vi "CSM-FileSync.vi"(5 "Name(FileSync)":string="FileSync", 7 "Protocol.lvclass":refnum<class "Protocol.lvclass">, 11 "FileSync Configuration":T1={"MonitoringFolder"=path "_sync/Monitoring", "BackupFolder"=path "_sync/backup", "autostart"=TRUE, "Backup"=FALSE}) -> (0 "error out":errorcluster)   [LabVIEW 2020, in "CSM-FileSync.lvlib"]
doc: "------------- lvcsm -------------\n[CSMStates]\nItem 0 = \"Idle\"\nItem 1 = \"Timeout\"\nItem 2 = \"Initialize Core Data\"\nItem 3 = \"Error Handler\"\nItem 4 = \"VI Reference\"\nItem 5 = \"Exit\"\nItem 6 = \"Data: Initialize\"\nItem 7 = \"Data: Load Configuration\"\nItem 8 = \"Data: Save Configuration\"\nItem 9 = \"Data: Cleanup\"\nItem 10 = \"UI: Initialize\"\nItem 11 = \"UI: Publish Status\"\nItem 12 = \"Macro: Initialize\"\nItem 13 = \"Macro: FileSync Protocol Connect\"\nItem 14 = \"Macro: Check Is Still Alive\"\nItem 15 = \"Macro: FileSync Routines\"\nItem 16 = \"Macro: FileSync Protocol Disconnect\"\nItem 17 = \"Macro: Exit\"\nItem 18 = \"API: Start\"\nItem 19 = \"API: Stop\"\nItem 20 = \"FileSync: Load Configuration\"\nItem 21 = \"FileSync: Try to Connect\"\nItem 22 = \"FileSync: Status Check\"\nItem 23 = \"FileSync: Close Connection\"\nItem 24 = \"FileSync: Cleanup Protocol\"\nItem 25 = \"FileSyncRoutine: Create Dir if Not Exist\"\nItem 26 = \"FileSyncRoutine: List Files\"\nItem 27 = \"FileSyncRoutine: Pick Uploading File\"\nItem 28 = \"FileSyncRoutine: Upload\"\nItem 29 = \"FileSyncRoutine: Move File to Backup Folder\"\nItem 30 = \"FileSyncRoutine: Remove Empty Container Folder\"\n\n[CSMStatus]\nItem 0 = \"Status Change@UI: Publish Status\"\nItem 1 = \"Uploading List Change@UI: Publish Status\""
uses:
  CSM-FileSync.lvlib
  Protocol/Base/Protocol.lvclass
  Protocol/Base/Def-FileSyncConfig.ctl
  c11ad69d-c218-40bd-9883-d3361c9d07ec.vi
  4f3a877e-8c3a-40cf-89f4-fda6eeae6ffa.vi
  d714c97a-ade9-4c5a-b010-05319b638c8a.vi
  16b40464-5854-4f01-88e3-2a837e9228b3.vi
  16b40464-5854-4f01-88e3-2a837e9228b3.vi/eb2405bd-5b2e-436b-9bb3-692ecf4a9268.vi
  16b40464-5854-4f01-88e3-2a837e9228b3.vi/c8ad12e3-5e6d-40e1-92e0-1426ef45ec41.vi
  16b40464-5854-4f01-88e3-2a837e9228b3.vi/effcbc1a-e97c-42d4-b61f-d821de102707.vi
  <userlib>/_NEVSTOP/Communicable State Machine(CSM)/addons/MassData-Parameter/_support/FGV-MassData(lvlibp).vi
  <userlib>/_NEVSTOP/Communicable State Machine(CSM)/_Polymophic/Add State(s) to Queue By BOOL(Element).vi
  <userlib>/_NEVSTOP/Communicable State Machine(CSM)/_Polymophic/Build Status Broadcast Message.vi
  <userlib>/_NEVSTOP/Communicable State Machine(CSM)/AdvanceAPI/CSM - Set Module Attribute.vi
  <userlib>/_NEVSTOP/Communicable State Machine(CSM)/addons/API-String-Arugments-Support/_Support/Data To API String Arguments.vi
  <userlib>/_NEVSTOP/Communicable State Machine(CSM)/Communicable State Machine.lvlib
  <userlib>/_NEVSTOP/Communicable State Machine(CSM)/addons/Logger/CSM File Logger.lvlib
  <userlib>/_NEVSTOP/Communicable State Machine(CSM)/addons/Loop-Support/CSM Loop Support.lvlib
  <userlib>/_NEVSTOP/Communicable State Machine(CSM)/addons/MassData-Parameter/CSM MassData Parameter Support.lvlib
panel:
  out "State History":string
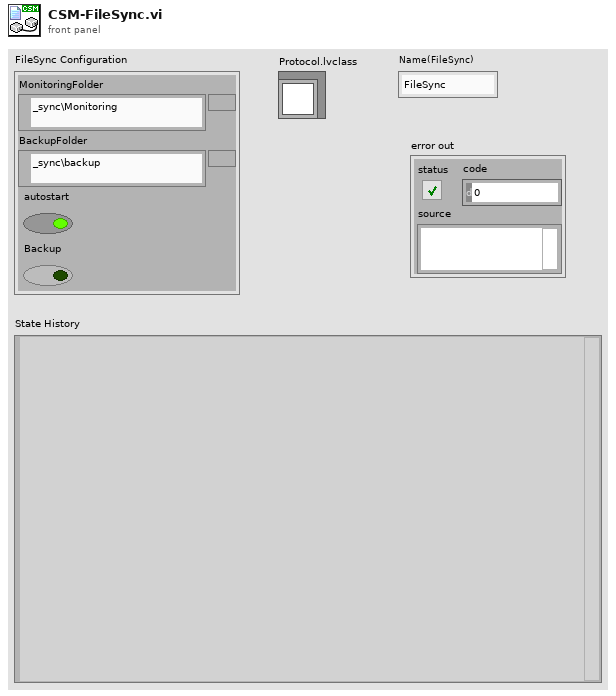
[diagram p1: front panel]
types:
  T1 = typedef "CSM-FileSync.lvlib/Protocol.lvclass/Def-FileSyncConfig.ctl" = cluster{"MonitoringFolder":path, "BackupFolder":path, "autostart":bool, "Backup":bool}
  T2 = enum32{"Invalid", "Standard", "Closed", "Hidden", "Minimized", "Maximized"}
  T3 = enum32{"invalid app kind", "Development System", "Run Time System", "Student Edition", "Embedded LabVIEW", "Evaluation", "Custom"}
  T4 = cluster{"Upload List":path[], "UploadingFile":path}
  T5 = typedef "Communicable State Machine.lvlib/_CSM_Response Source Message.ctl" = cluster{"‘State":string, "’Arguments":string, "’Error":errorcluster}
  T6 = cluster{"Core":cluster{"Current VI Reference":refnum<vi>, "Close Panel on Exit?":bool}, "Configuration":T1, "FileSync Status":cluster{"Connected":bool}, "Upload List":path[], "Temp:UploadingFile":path}
  T7 = cluster{"Current VI Reference":refnum<vi>, "Close Panel on Exit?":bool}
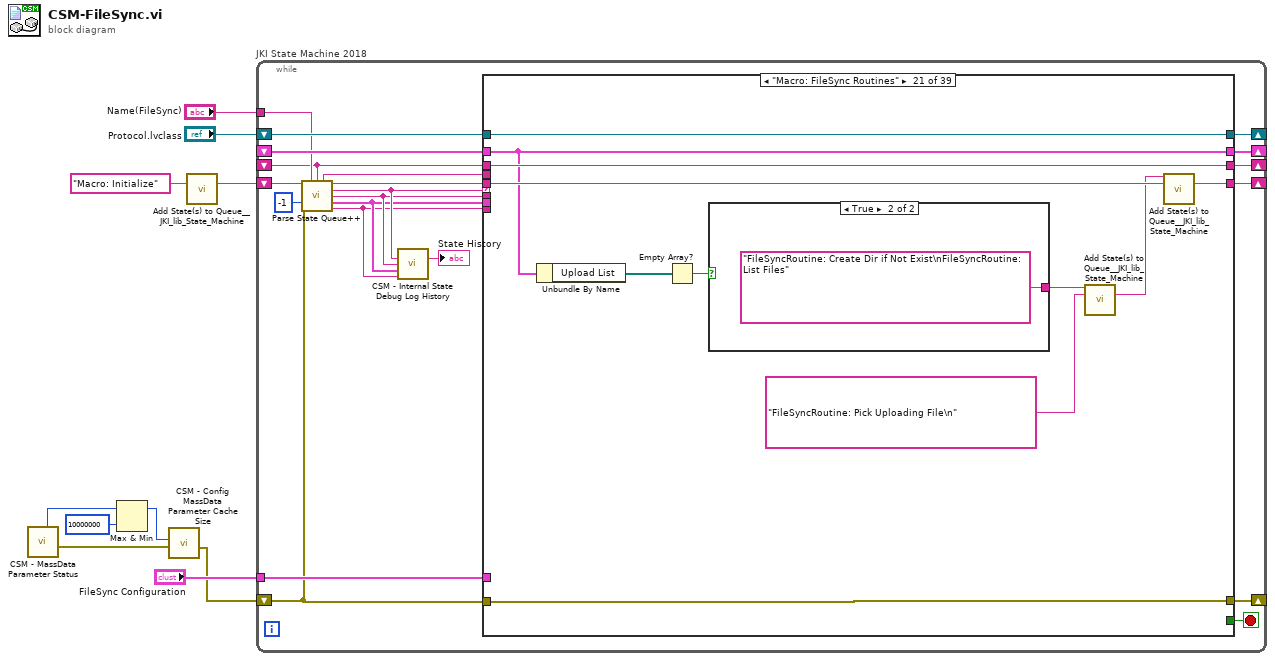
[diagram p0: block diagram]
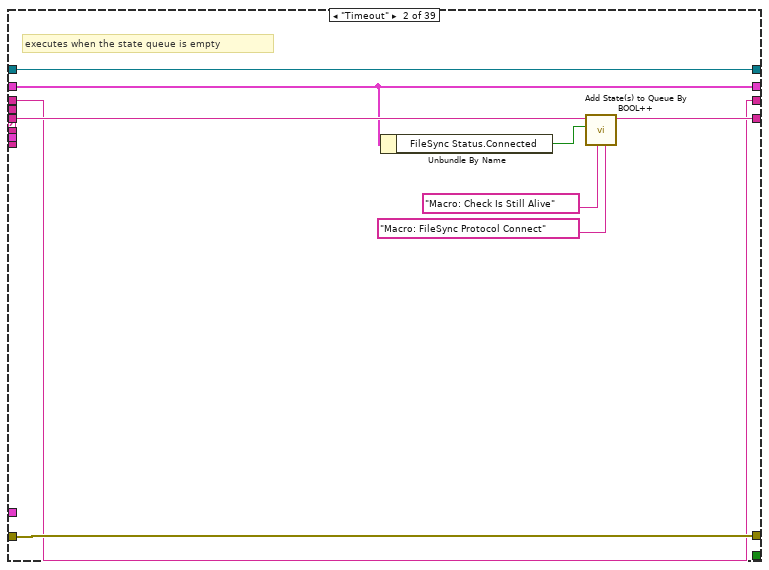
[diagram p3: hidden frame]
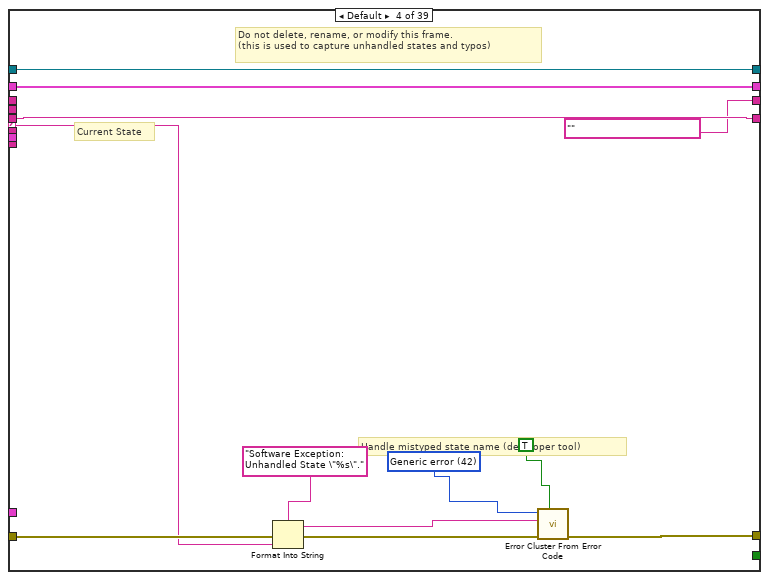
[diagram p5: hidden frame]
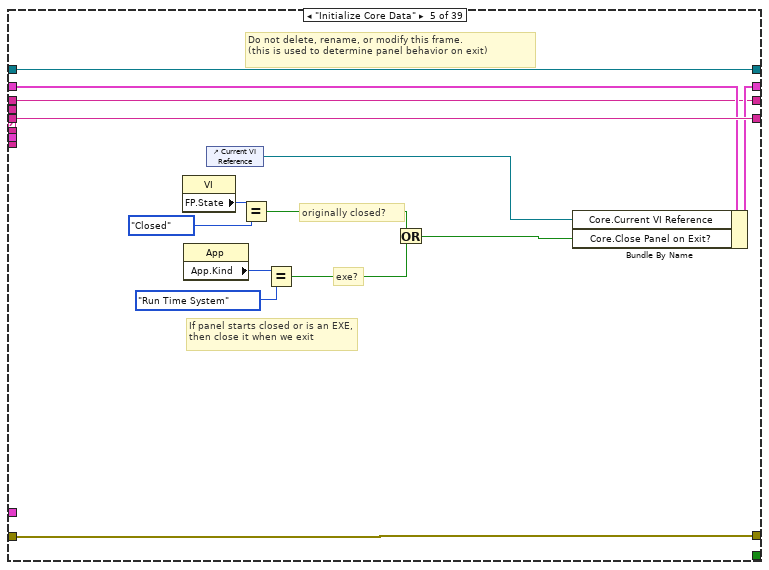
[diagram p6: hidden frame]
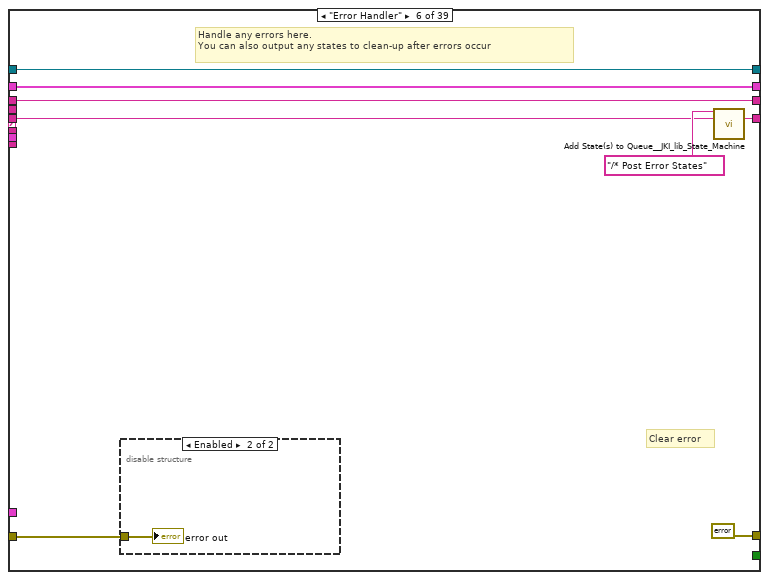
[diagram p7: hidden frame]
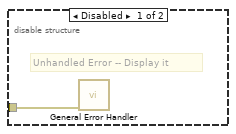
[diagram p8: hidden frame]
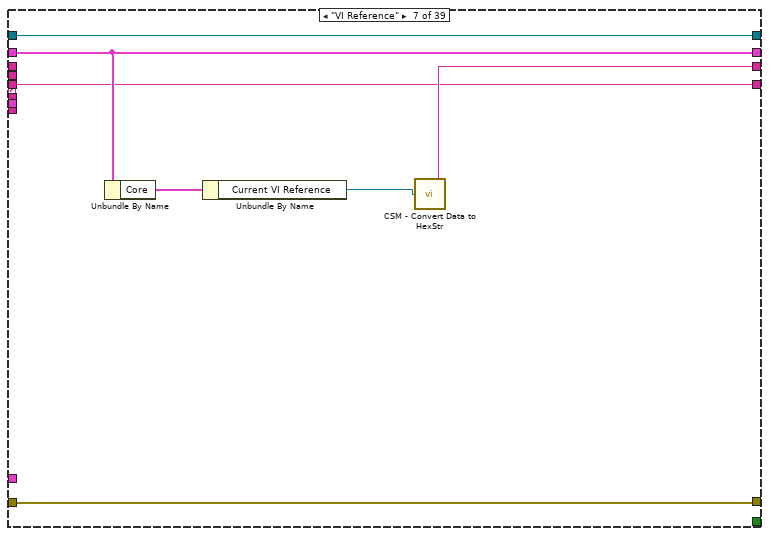
[diagram p9: hidden frame]
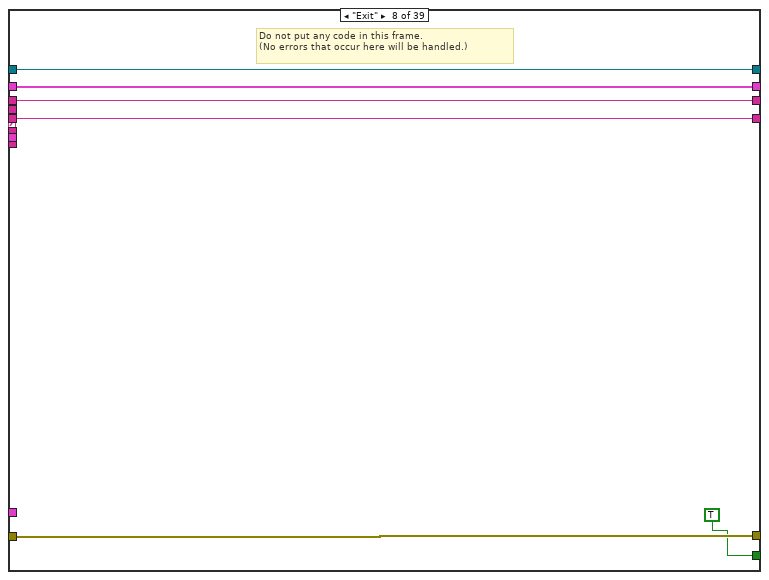
[diagram p10: hidden frame]
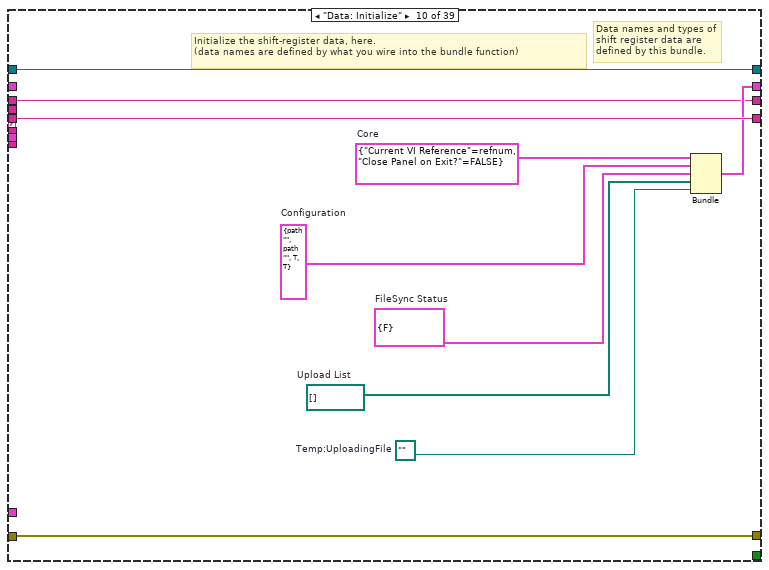
[diagram p12: hidden frame]
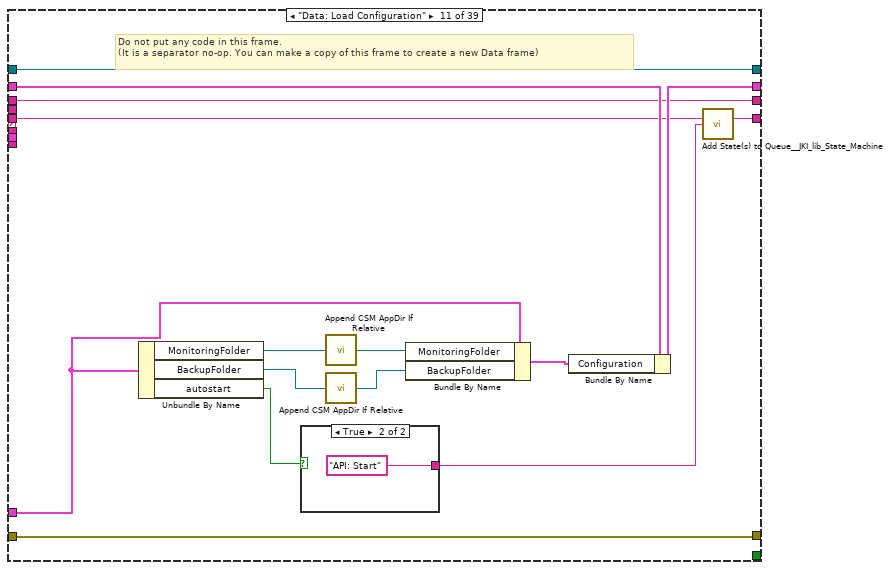
[diagram p13: hidden frame]
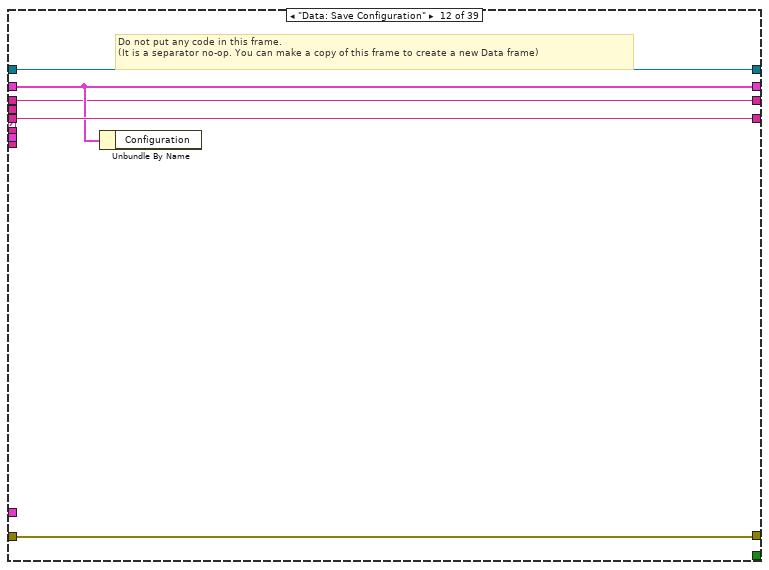
[diagram p15: hidden frame]
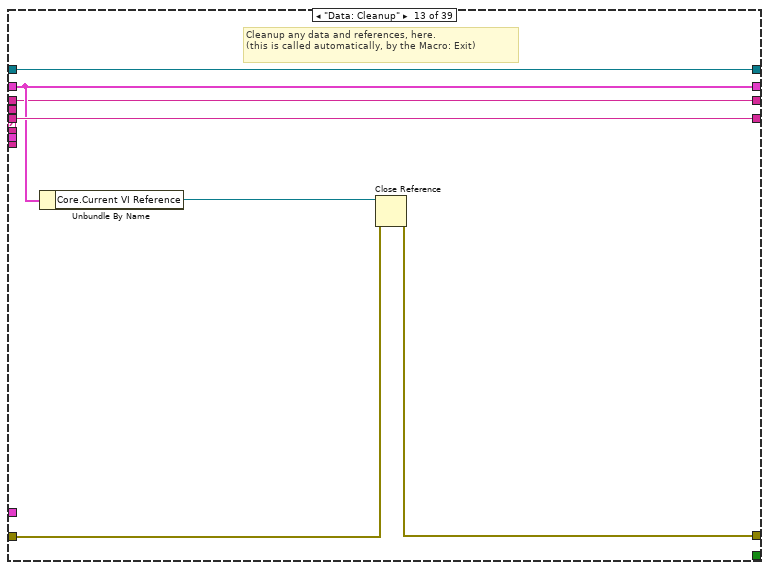
[diagram p16: hidden frame]
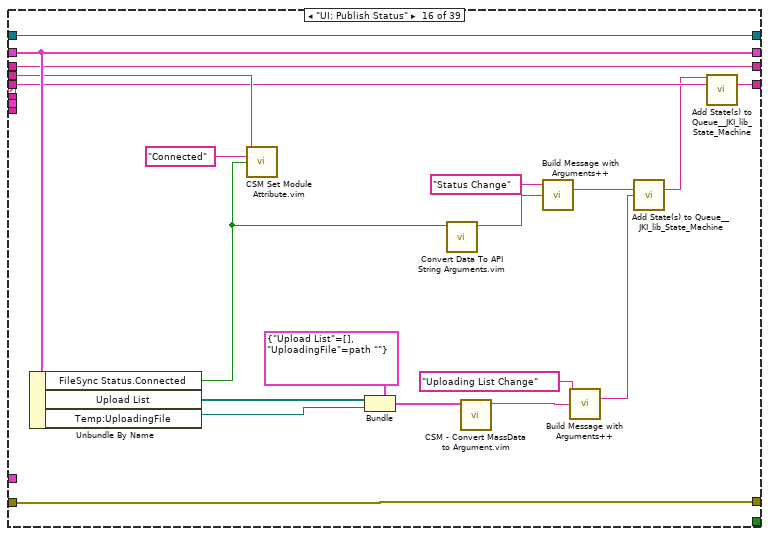
[diagram p19: hidden frame]
diagram:
  n1 = call <userlib>:"CSM - MassData Parameter Status.vi"() -> ("Error out"=w5:errorcluster, "Cache Size"=w2:i32)  [unwired: 7 in, 2 out]
  n2 = Max & Min(x=w2, y=10000000) -> (max(x,y)=w3:i32)  [unwired: 1 out]
  n3 = call <userlib>:"CSM - Config MassData Parameter Cache Size.vi"("Error in"=w5, "Size (50M)"=w3) -> ("Error out"=w4:errorcluster)  [unwired: 9 in]
  n4 = call <vilib>:"Add State(s) to Queue__JKI_lib_State_Machine.vi"("State(s) in (\"\")"="Macro: Initialize") -> ("States Out"=w10:string)  [unwired: 14 in]
  n5 = while "JKI State Machine 2018" {
    shift-right: [w28] -> _
    shift-left: _ -> [w27]
    shift-right: [w31] -> _
    shift-left: w4 -> [w22]
    shift-right: [w30] -> _
    shift-left: w10 -> [w23]
    shift-right: [w25] -> _
    shift-left: "Protocol.lvclass" -> [w26]
    tunnel: "FileSync Configuration" -> [w24]
    shift-right: [w20] -> _
    shift-left: _ -> [w17]
    tunnel: "Name(FileSync)" -> [w19]
    stop <- w29 stop-if-true
    n6 = call <userlib>:"Parse State Queue++.vi"("State Queue"=w23, "Name (\"\" to Use UUID)"=w19, "Response Arguments"=w17, "Previous Error"=w22, "Dequeue (1 ms)"=-1 ("Dequeue Timeout(1ms)")) -> ("Name Used"=w18:string, "Remaining States"=w21:string, "Current State"=w15:string, "Arguments"=w14:string, "Additional Information"=w13:T5, "Source CSM"=w12:string)  [unwired: 5 in]
    n7 = call <userlib>:"CSM - Internal State Debug Log History.vi"("State"=w15, "Arguments (\"\")"=w14, ">> Response Source Message >>"=w13, "Source (\"\")"=w12) -> ("Debug Log"=→"State History":string)  [unwired: 11 in]
    n8 = case shown="\"Macro: FileSync Routines\"" w15 {
      selector: w15 -> [_ _ _ w53 _ _ _ _ _ _ _ _ _ _ _ _ _ _ _ _ _ _ _ _ _ _ _ _ _ w274 _ _ _ _ _ _ _ _ _]
      tunnel: w21 -> [w32 w45 w50 w56 w76 w77 w89 w99 w104 w114 w118 w135 w142 w147 w152 w165 w177 w184 w189 w197 w208 w217 w233 w236 w242 w247 w253 w260 w269 w275 w292 w299 w304 w312 w321 w337 w347 w373 w415]
      tunnel: w14 -> [_ _ _ _ _ _ _ _ _ _ _ _ _ _ _ _ _ _ _ _ _ _ _ _ _ _ _ _ _ _ _ _ _ _ _ _ w355 w364 w409]
      tunnel: w27 -> [w35 w42 w48 w55 w70 w82 w93 w98 w102 _ w127 w133 w138 w145 w151 w170 w175 w181 w187 w195 w206 w215 w230 w235 w241 w246 w251 w259 w268 w279 w291 w298 w302 w309 w319 w333 w352 w371 w411]
      tunnel: [w36 w43 w49 w58 w74 errorcluster {"status"=FALSE, "code"=0, "source"=""} ("error out") w88 w97 w103 w112 w126 w132 w139 w146 w150 w171 w176 w182 w191 w199 w210 w219 w231 w237 w243 w248 w252 w257 w264 w282 w289 w296 w303 w305 w317 w335 w339 w368 w412] -> w31
      tunnel: w22 -> [w36 w43 w49 w57 w74 w81 w88 w97 w103 w112 w126 w132 w140 w146 w150 w171 w176 w182 w191 w199 w210 w219 w231 w237 w243 w248 w252 w258 w265 w283 w290 w297 w303 _ w316 w335 w353 _ w413]
      tunnel: [w32 w44 w50 w56 w76 w84 w89 w99 w104 w114 w119 w135 w142 w147 w152 w166 w177 w183 w190 w198 w209 w218 w232 w236 w239 w244 w253 w260 w269 w276 w292 w299 w304 w312 w321 w336 w348 w373 w415] -> w30
      tunnel: [_ _ _ _ _ _ _ TRUE _ _ _ _ _ _ _ _ _ _ _ _ _ _ _ _ _ _ _ _ _ _ _ _ _ _ _ _ _ _ _] -> w29
      tunnel: [w35 w42 w48 w55 w75 w82 w93 w98 w102 w113 w128 w133 w138 w145 w151 w170 w175 w181 w187 w195 w206 w215 w230 w235 w241 w246 w251 w259 w263 w279 w286 w298 w302 w309 w315 w332 w352 w365 w411] -> w28
      tunnel: w26 -> [w34 w41 w47 w52 w64 w79 w87 w95 w101 w110 w129 w134 w137 w144 w149 w172 w174 w179 w192 w200 w211 w220 w223 w234 w240 w245 w250 w256 w267 w281 w288 w295 w301 w311 w320 w334 w350 w372 w414]
      tunnel: [w34 w41 w47 w52 w64 w79 w87 w95 w101 w110 w129 w134 w137 w144 w149 w172 w174 w179 w192 w200 w211 w220 w223 w234 w240 w245 w250 w255 w266 w280 w287 w294 w301 w311 w320 w334 w354 w372 w414] -> w25
      tunnel: w24 -> [_ _ _ _ _ _ _ _ _ _ w115 _ _ _ _ _ _ _ _ _ _ _ _ _ _ _ _ _ _ _ _ _ _ _ _ _ _ _ _]
      tunnel: [w33 w40 w46 "" ("message") w63 w78 w90 w94 w100 w105 w124 w131 w136 w143 w148 w169 w173 w178 w185 w194 w207 w213 w222 _ _ _ w249 w254 w261 w278 w284 w293 w300 w306 w313 w325 w349 w367 w406] -> w20
      tunnel: w12 -> [_ _ _ _ _ _ _ _ _ _ _ _ _ _ _ _ _ _ _ _ _ _ _ _ _ _ _ _ _ _ _ _ _ _ _ _ _ _ _]
      tunnel: w13 -> [_ _ _ _ _ _ _ _ _ _ _ _ _ _ _ _ _ _ _ _ _ _ _ _ _ _ _ _ _ _ _ _ _ _ _ _ _ _ _]
      tunnel: w18 -> [_ _ _ _ _ _ _ _ _ _ _ _ _ _ _ w168 _ _ _ _ _ _ _ _ _ _ _ _ _ _ _ _ _ _ _ _ _ _ _]
      tunnel: w17 -> [w33 w40 w46 _ w63 w78 _ w94 w100 w105 w124 w131 w136 w143 w148 w169 w173 w178 w185 w194 w207 w213 w222 _ _ _ w249 w254 w261 w278 w284 w293 w300 w306 w313 w325 w349 w367 w406]
      frame "", "Idle" {
      }
      frame "Timeout" {
        # "executes when the state queue is empty"
        n9 = Unbundle By Name(w42) -> ("FileSync Status.Connected"=w37:bool)
        n10 = call-poly <userlib>:"Add State(s) to Queue By BOOL++.vi"("FALSE (\"\")"="Macro: FileSync Protocol Connect" ("State(s) in Front (\"\")"), "TRUE (\"\")"="Macro: Check Is Still Alive" ("State(s) in Front (\"\")"), "Condition"=w37, "State Queue (\"\")"=w45) -> ("Remaining States"=w44:string)  [unwired: 7 in]
      }
      frame "---------- Core ----------" {
        # "Do not put any code in this frame.\n(it is a separator no-op)"
      }
      frame Default {
        w61 = 42 items=["No error", "Argument error", "Memory is full", "Out of zone", "End of file", "File already open", "Generic file I/O error", "File not found", "File permission error", "Disk is full", "Duplicate path", "Too many files open", "System feature not enabled", "Resource file not found", "Cannot add resource", "Resource not found", "Image not found", "Image memory error", "Pen does not exist", "Config type invalid", "Config token not found", "Config parse error", "Config memory error", "Bad external code format", "Bad external code offset", "External code not present", "Null window", "Destroy window error", "Null menu", "Print aborted", "Bad print record", "Print driver error", "Windows error during printing", "Memory error during printing", "Print dialog error", "Generic print error", "Invalid device refnum", "Device not found", "Device parameter error", "Device unit error", "Cannot open device", "Device call aborted", "Generic error", "Cancelled by user", "Object ID too low", "Object ID too high", "Object not in heap", "Unknown heap", "Unknown object (invalid DefProc)", "Unknown object (DefProc not in table)", "Message out of range", "Invalid (null) method", "Unknown message", "Manager call not supported", "Bad address", "Network operation in progress", "Network operation timed out", "Connection is busy", "Network attribute not supported", "Network error", "Address in use", "System out of memory", "Connection aborted", "Connection refused", "Not connected", "Already connected", "Connection closed", "Initialization error (interapplication manager)", "Bad occurrence", "Wait on unbound occurrence handler", "Occurrence queue overflow", "Datalog type conflict", "Unused", "Unrecognized type (interapplication manager)", "Memory corrupt", "Failed to make temporary DLL", "Old CIN version", "Drag socket not found", "Failed to load drop-object", "Failed to register OLE object", "Failed to release OLE object", "Format specifier type mismatch", "Unknown format specifier", "Too few format specifiers", "Too many format specifiers", "Scan failed", "Newer CIN version", "Error converting to variant", "Runtime menu error", "Password tampered", "Variant attribute not found", "Incompatible variant data type", "Event data is not available", "Event Store is not present", "Occurrence is not found", "Event Queue is not created", "Event info is not available", "Refnum passed is NULL", "Error retrieving Class GUID", "Error retrieving CoClass GUID", "Error retrieving TypeLib GUID.", "Bad built application magic bytes.", "Specific driver is different from the specific driver associated with the Logical Name.", "There is no session opened to the class driver.", "Max Error", "MAX - Error with config objects", "MAX - Error loading configuration", "MAX - Group not supported"]
        # "Current State"
        # "Do not delete, rename, or modify this frame.\n(this is used to capture unhandled states and typos)"
        # "Handle mistyped state name (developer tool)"
        n11 = Format Into String(format string="Software Exception: Unhandled State \"%s\"." ("message"), error in=w57, w53) -> (resulting string=w60:string, error out=w59:errorcluster)  [unwired: 1 in]
        n12 = call <vilib>:"Error Cluster From Error Code.vi"("show call chain? (False)"=TRUE, "error in (no error)"=w59, "error message (\"\")"=w60, "error code (0)"=w61) -> ("error out"=w58:errorcluster)  [unwired: 5 in]
      }
      frame "Initialize Core Data" {
        # "Do not delete, rename, or modify this frame.\n(this is used to determine panel behavior on exit)"
        # "originally closed?"
        # "exe?"
        # "If panel starts closed or is an EXE, then close it when we exit"
        n13 = property class="VI"() -> ("FP.State"=w67:T2)  [unwired: 2 in, 2 out]
        n14 = property class="App"() -> ("App.Kind"=w73:T3)  [unwired: 2 in, 2 out]
        n15 = control-ref of="Current VI Reference"() -> (w68:refnum<vi>)
        n16 = Equal?(x=w67, y=T2."Closed" ("Front Panel Window:State")) -> (x = y?=w65:bool)
        n17 = Equal?(x=w73, y=T3."Run Time System" ("Application:Kind")) -> (x = y?=w71:bool)
        n18 = Or(x=w65, y=w71) -> (x .or. y?=w69:bool)
        n19 = Bundle By Name(cluster=w70, "Core.Current VI Reference"=w68, "Core.Close Panel on Exit?"=w69) -> (w75:T6)
      }
      frame "Error Handler" {
        # "Handle any errors here.\nYou can also output any states to clean-up after errors occur"
        # "Clear error"
        n20 = disable-structure shown="Enabled" {
          disable-tunnel: w81 -> [w85 w86]
          frame Disabled {
            # "Unhandled Error -- Display it"
            n21 = call <vilib>:"General Error Handler.vi"("error in (no error)"=w85) -> ()  [unwired: 10 in, 5 out]
          }
          frame Enabled {
            "error out" <- w86
          }
        }
        n22 = call <vilib>:"Add State(s) to Queue__JKI_lib_State_Machine.vi"("State(s) in Front (\"\")"="/* Post Error States", "State(s) in (\"\")"=w77) -> ("States Out"=w84:string)  [unwired: 13 in]
      }
      frame "VI Reference" {
        n23 = Unbundle By Name(w93) -> ("Core"=w92:T7)
        n24 = Unbundle By Name(w92) -> ("Current VI Reference"=w91:refnum<vi>)
        n25 = call <userlib>:"CSM - Convert Data to HexStr.vi"("Variant"=w91) -> ("HEX String (0-9,A-F)"=w90:string)  [unwired: 8 in]
      }
      frame "Exit" {
        # "Do not put any code in this frame.\n(No errors that occur here will be handled.)"
      }
      frame "---------- Data ----------" {
        # "Do not put any code in this frame.\n(It is a separator no-op. You can make a copy of this frame to create a new Data frame)"
      }
      frame "Data: Initialize" {
        w106 = path ""  # Temp:UploadingFile
        w107 = path[] []  # Upload List
        w108 = cluster{"Connected":bool} {"Connected"=FALSE}  # FileSync Status
        w109 = T1 {"MonitoringFolder"=path "", "BackupFolder"=path "", "autostart"=TRUE, "Backup"=TRUE}  # Configuration
        w111 = T7 {"Current VI Reference"=refnum, "Close Panel on Exit?"=FALSE}  # Core
        # "Data names and types of shift register data are defined by this bundle."
        # "Initialize the shift-register data, here.\n(data names are defined by what you wire into the bundle function)"
        n26 = Bundle("Core"=w111, "Configuration"=w109, "FileSync Status"=w108, "Upload List"=w107, "Temp:UploadingFile"=w106) -> (w113:T6)  [unwired: 1 in]
      }
      frame "Data: Load Configuration" {
        # "Do not put any code in this frame.\n(It is a separator no-op. You can make a copy of this frame to create a new Data frame)"
        n27 = Unbundle By Name(w115) -> ("MonitoringFolder"=w123:path, "BackupFolder"=w122:path, "autostart"=w116:bool)
        n28 = case shown="True" w116 {
          tunnel: [_ "API: Start" ("State(s) at Back (\"\")")] -> w117
          frame False {
          }
          frame True {
          }
        }
        n29 = call <userlib>:"Append CSM AppDir If Relative.vi"("Relative Path (.)"=w123) -> ("Application Directory (+ Relative)"=w121:path)  [unwired: 4 in]
        n30 = call <userlib>:"Append CSM AppDir If Relative.vi"("Relative Path (.)"=w122) -> ("Application Directory (+ Relative)"=w120:path)  [unwired: 4 in]
        n31 = Bundle By Name(cluster=w115, "MonitoringFolder"=w121, "BackupFolder"=w120) -> (w125:T1)
        n32 = Bundle By Name(cluster=w127, "Configuration"=w125) -> (w128:T6)
        n33 = call <vilib>:"Add State(s) to Queue__JKI_lib_State_Machine.vi"("State(s) in (\"\")"=w118, "State(s) at Back (\"\")"=w117) -> ("States Out"=w119:string)  [unwired: 13 in]
      }
      frame "Data: Save Configuration" {
        # "Do not put any code in this frame.\n(It is a separator no-op. You can make a copy of this frame to create a new Data frame)"
        n34 = Unbundle By Name(w133) -> ()  [unwired: 1 out]
      }
      frame "Data: Cleanup" {
        # "Cleanup any data and references, here.\n(this is called automatically, by the Macro: Exit)"
        n35 = Unbundle By Name(w138) -> ("Core.Current VI Reference"=w141:refnum<vi>)
        n36 = Close Reference(reference=w141, error in (no error)=w140) -> (error out=w139:errorcluster)
      }
      frame "---------- UI ----------" {
        # "Do not put any code in this frame.\n(It is a separator no-op. You can make a copy of this frame to create a new UI frame)"
      }
      frame "UI: Initialize" {
      }
      frame "UI: Publish Status" {
        n37 = Unbundle By Name(w170) -> ("FileSync Status.Connected"=w164:bool, "Upload List"=w153:path[], "Temp:UploadingFile"=w163:path)
        n38 = call "CSM Set Module Attribute.vim"("CSM Name"=w168, "Attribute"="Connected", "Value"=w164) -> ()  [unwired: 9 in, 4 out]
        n39 = Bundle(cluster=T4 {"Upload List"=[], "UploadingFile"=path ""} ("output cluster"), "Upload List"=w153, "UploadingFile"=w163) -> (w161:T4)
        n40 = call "Convert Data To API String Arguments.vim"("Data"=w164) -> ("API String"=w154:string)  [unwired: 7 in, 1 out]
        n41 = call "CSM - Convert MassData to Argument.vim"("Data"=w161) -> ("MassData Argument"=w156:string)  [unwired: 7 in, 1 out]
        n42 = call-poly <userlib>:"Build Message with Arguments++.vi"("State With Arguments"="Status Change" ("Attribute"), "Arguments (\"\")"=w154) -> ("CSM Message String"=w160:string)  [unwired: 13 in]
        n43 = call-poly <userlib>:"Build Message with Arguments++.vi"("State With Arguments"="Uploading List Change" ("Attribute"), "Arguments (\"\")"=w156) -> ("CSM Message String"=w159:string)  [unwired: 13 in]
        n44 = call <vilib>:"Add State(s) to Queue__JKI_lib_State_Machine.vi"("State(s) in (\"\")"=w160, "State(s) at Back (\"\")"=w159) -> ("States Out"=w158:string)  [unwired: 13 in]
        n45 = call <vilib>:"Add State(s) to Queue__JKI_lib_State_Machine.vi"("State(s) in Front (\"\")"=w158, "State(s) in (\"\")"=w165) -> ("States Out"=w166:string)  [unwired: 13 in]
      }
      frame "---------- Macro ----------" {
        # "Do not put any code in this frame.\n(It is a separator no-op. You can make a copy of this frame to create a new Macro frame)"
      }
      frame "Macro: Initialize" {
        # "Initialization Macro\n(This is called once, when the VI starts)"
        n46 = call <vilib>:"Add State(s) to Queue__JKI_lib_State_Machine.vi"("State(s) in Front (\"\")"="Data: Initialize\nInitialize Core Data\nData: Load Configuration\nUI: Initialize\nUI: Publish Status\n//UI: Front Panel State >> Open\n", "State(s) in (\"\")"=w184) -> ("States Out"=w183:string)  [unwired: 13 in]
      }
      frame "Macro: FileSync Protocol Connect" {
        n47 = Unbundle By Name(w187) -> ("FileSync Status.Connected"=w186:bool)
        n48 = case shown="True" w186 {
          tunnel: [_ "FileSync: Load Configuration\nFileSync: Try to Connect\nUI: Publish Status" ("State(s) in Front (\"\")")] -> w188
          frame False {
          }
          frame True {
          }
        }
        n49 = call <vilib>:"Add State(s) to Queue__JKI_lib_State_Machine.vi"("State(s) in Front (\"\")"=w188, "State(s) in (\"\")"=w189) -> ("States Out"=w190:string)  [unwired: 13 in]
      }
      frame "Macro: Check Is Still Alive" {
        n50 = call <vilib>:"Add State(s) to Queue__JKI_lib_State_Machine.vi"("State(s) in Front (\"\")"="FileSync: Check Connection is Still Alive" ("State(s) in Front (\"\")"), "State(s) in (\"\")"=w197) -> ("States Out"=w198:string)  [unwired: 13 in]
      }
      frame "Macro: FileSync Routines" {
        n51 = Unbundle By Name(w206) -> ("Upload List"=w205:path[])
        n52 = Empty Array?(array=w205) -> (empty?=w201:bool)
        n53 = case shown="True" w201 {
          tunnel: [_ "FileSyncRoutine: Create Dir if Not Exist\nFileSyncRoutine: List Files" ("State(s) in Front (\"\")")] -> w204
          frame False {
          }
          frame True {
          }
        }
        n54 = call <vilib>:"Add State(s) to Queue__JKI_lib_State_Machine.vi"("State(s) in Front (\"\")"=w204, "State(s) in (\"\")"="FileSyncRoutine: Pick Uploading File\n" ("State(s) in Front (\"\")")) -> ("States Out"=w202:string)  [unwired: 13 in]
        n55 = call <vilib>:"Add State(s) to Queue__JKI_lib_State_Machine.vi"("State(s) in Front (\"\")"=w202, "State(s) in (\"\")"=w208) -> ("States Out"=w209:string)  [unwired: 13 in]
      }
      frame "Macro: FileSync Protocol Disconnect" {
        n56 = Unbundle By Name(w215) -> ("FileSync Status.Connected"=w214:bool)
        n57 = case shown="True" w214 {
          tunnel: [_ "FileSync: Close Connection\nFileSync: Cleanup Protocol\nUI: Publish Status" ("State(s) in Front (\"\")")] -> w216
          frame False {
          }
          frame True {
          }
        }
        n58 = call <vilib>:"Add State(s) to Queue__JKI_lib_State_Machine.vi"("State(s) in Front (\"\")"=w216, "State(s) in (\"\")"=w217) -> ("States Out"=w218:string)  [unwired: 13 in]
      }
      frame "Macro: Exit" {
        # "Exit Macro\n(This is called once, when the VI exits)"
        n59 = Unbundle By Name(w230) -> ("Core.Close Panel on Exit?"=w229:bool)
        n60 = Select(t="//UI: Front Panel State >> Close", s=w229, f="") -> (s? t:f=w226:string)
        n61 = call <vilib>:"Add State(s) to Queue__JKI_lib_State_Machine.vi"("State(s) in (\"\")"=w226, "State(s) at Back (\"\")"="Macro: FileSync Protocol Disconnect\nData: Cleanup\nExit") -> ("States Out"=w224:string)  [unwired: 13 in]
        n62 = call <vilib>:"Add State(s) to Queue__JKI_lib_State_Machine.vi"("State(s) in Front (\"\")"=w224, "State(s) in (\"\")"=w233) -> ("States Out"=w232:string)  [unwired: 13 in]
      }
      frame "---------- API ----------" {
      }
      frame "API: Start" {
        n63 = call <userlib>:"CSMLS - Define Loop State(s).vi"("Loop States"="FileSync: Load Configuration\nFileSync: Try to Connect\nFileSync: Status Check -><loop>\nFileSync: Close Connection\nFileSync: Cleanup Protocol" ("Loop State(s) and Arguments"), "States Queue"=w242) -> ("Remaining States"=w239:string)  [unwired: 13 in]
      }
      frame "API: Stop" {
        n64 = call <userlib>:"CSMLS - Remove Loop Tag and previous State(s) to Break.vi"("States Queue"=w247) -> ("Remaining States"=w244:string)  [unwired: 10 in]
      }
      frame "---------- FileSync ----------" {
      }
      frame "FileSync: Load Configuration" {
        n65 = call-dynamic "Initialize.vi"("error in (no error)"=w258, "Protocol in"=w256) -> ("error out"=w257:errorcluster, "Protocol out"=w255:refnum<class "Protocol.lvclass">)  [unwired: 8 in]
      }
      frame "FileSync: Try to Connect" {
        n66 = call-dynamic "Connect.vi"("error in (no error)"=w265, "Protocol in"=w267) -> ("error out"=w264:errorcluster, "Connected?"=w262:bool, "Protocol out"=w266:refnum<class "Protocol.lvclass">)  [unwired: 7 in]
        n67 = Bundle By Name(cluster=w268, "FileSync Status.Connected"=w262) -> (w263:T6)
      }
      frame "FileSync: Status Check" {
        n68 = call-dynamic "Check.vi"("error in (no error)"=w283, "Protocol in"=w281) -> ("error out"=w282:errorcluster, "Still alive?"=w277:bool, "Protocol out"=w280:refnum<class "Protocol.lvclass">)  [unwired: 7 in]
        n69 = Select(t="Macro: FileSync Routines" ("State(s) in Front (\"\")"), s=w277, f="Macro: FileSync Protocol Disconnect\nFileSync: Load Configuration\nFileSync: Try to Connect" ("State(s) in Front (\"\")")) -> (s? t:f=w272:string)
        n70 = Wait (ms)(milliseconds to wait=u32 200) -> ()  [unwired: 1 out]
        n71 = call <userlib>:"CSMLS - Append Continuous State.vi"("Loop State(s) And Arguments"=w272, "Continous State"=w274, "States Queue"=w275) -> ("Remaining States"=w276:string)  [unwired: 8 in]
      }
      frame "FileSync: Close Connection" {
        n72 = call-dynamic "Disconnect.vi"("error in (no error)"=w290, "Protocol in"=w288) -> ("error out"=w289:errorcluster, "Protocol out"=w287:refnum<class "Protocol.lvclass">)  [unwired: 8 in]
        n73 = Bundle By Name(cluster=w291, "FileSync Status.Connected"=FALSE) -> (w286:T6)
      }
      frame "FileSync: Cleanup Protocol" {
        n74 = call-dynamic "Cleanup.vi"("error in (no error)"=w297, "Protocol in"=w295) -> ("error out"=w296:errorcluster, "Protocol out"=w294:refnum<class "Protocol.lvclass">)  [unwired: 8 in]
      }
      frame "---------- FileSyncRoutine ----------" {
      }
      frame "FileSyncRoutine: Create Dir if Not Exist" {
        n75 = Unbundle By Name(w309) -> ("Configuration.MonitoringFolder"=w308:path, "Configuration.BackupFolder"=w307:path)
        n76 = call <vilib>:"Create Directory Recursive.vi"("directory"=w308) -> ("error out"=w310:errorcluster)  [unwired: 4 in, 2 out]
        n77 = call <vilib>:"Create Directory Recursive.vi"("error in (no error)"=w310, "directory"=w307) -> ("error out"=w305:errorcluster)  [unwired: 3 in, 2 out]
      }
      frame "FileSyncRoutine: List Files" {
        n78 = Unbundle By Name(w319) -> ("Configuration.MonitoringFolder"=w318:path)
        n79 = call <vilib>:"Recursive File List.vi"("error in (no error)"=w316, "Folder Path"=w318) -> ("error out"=w317:errorcluster, "All Files in Dir"=w314:path[])  [unwired: 5 in, 3 out]
        n80 = Bundle By Name(cluster=w319, "Upload List"=w314) -> (w315:T6)
      }
      frame "FileSyncRoutine: Pick Uploading File" {
        n81 = Unbundle By Name(w333) -> ("Upload List"=w327:path[])
        n82 = Index Array(array=w327) -> (element=w326:path)  [unwired: 1 in]
        n83 = Path To String(path=w326) -> (string=w328:string)
        n84 = Bundle By Name(cluster=w333, "Temp:UploadingFile"=w326) -> (w332:T6)
        n85 = Empty String/Path?(string/path=w326) -> (empty?=w331:bool)
        n86 = call <vilib>:"Build State String with Arguments__JKI_lib_State_Machine.vi"("Arguments (\"\")"=w328, "State"="FileSyncRoutine: Upload" ("False(Empty)")) -> ("State with Arguments"=w323:string)  [unwired: 4 in]
        n87 = call <vilib>:"Add State(s) to Queue__JKI_lib_State_Machine.vi"("State(s) in Front (\"\")"="UI: Publish Status" ("False(Empty)"), "State(s) in (\"\")"=w323) -> ("States Out"=w330:string)  [unwired: 13 in]
        n88 = call-poly <userlib>:"Add State(s) to Queue By BOOL++.vi"("FALSE (\"\")"=w330, "High Priority? (F)"=TRUE ("High Priority(FALSE)"), "Condition"=w331, "State Queue (\"\")"=w337) -> ("Remaining States"=w336:string)  [unwired: 7 in]
      }
      frame "FileSyncRoutine: Upload" {
        n89 = String To Path(string=w355) -> (path=w340:path)
        n90 = Unbundle By Name(w352) -> ("Configuration.MonitoringFolder"=w351:path)
        n91 = call-dynamic "UploadFile.vi"("Root Path"=w351, "error in (no error)"=w353, "Path"=w340, "Protocol in"=w350) -> ("error out"=w339:errorcluster, "Protocol out"=w354:refnum<class "Protocol.lvclass">)  [unwired: 6 in]
        n92 = Path To String(path=w340) -> (string=w344:string)
        n93 = call <vilib>:"Build State String with Arguments__JKI_lib_State_Machine.vi"("Arguments (\"\")"=w344, "State"="FileSyncRoutine: Move File to Backup Folder" ("False(Empty)")) -> ("State with Arguments"=w345:string)  [unwired: 4 in]
        n94 = call <vilib>:"Build State String with Arguments__JKI_lib_State_Machine.vi"("Arguments (\"\")"=w344, "State"="FileSyncRoutine: Remove Empty Container Folder" ("False(Empty)")) -> ("State with Arguments"=w346:string)  [unwired: 4 in]
        n95 = case shown="No Error" w339 {
          tunnel: w346 -> [w357 _]
          tunnel: w345 -> [w358 _]
          tunnel: [w359 _] -> w341
          tunnel: "UI: Publish Status" ("False(Empty)") -> [w356 _]
          frame No Error {
            n96 = call <vilib>:"Add State(s) to Queue__JKI_lib_State_Machine.vi"("State(s) in Front (\"\")"=w358, "State(s) in (\"\")"=w357, "State(s) at Back (\"\")"=w356) -> ("States Out"=w359:string)  [unwired: 12 in]
          }
          frame Error {
          }
        }
        n97 = call <vilib>:"Add State(s) to Queue__JKI_lib_State_Machine.vi"("State(s) in Front (\"\")"=w341, "State(s) in (\"\")"=w347) -> ("States Out"=w348:string)  [unwired: 13 in]
      }
      frame "FileSyncRoutine: Move File to Backup Folder" {
        n98 = Unbundle By Name(w371) -> ("Upload List"=w363:path[], "Configuration.Backup"=w366:bool, "Configuration.BackupFolder"=w370:path, "Configuration.MonitoringFolder"=w369:path)
        n99 = String To Path(string=w364) -> (path=w362:path)
        n100 = case shown="True" w366 {
          tunnel: w370 -> [w378 w403]
          tunnel: w369 -> [w377 w402]
          tunnel: [w376 w401] -> w368
          tunnel: w362 -> [w374 w399]
          frame True {
            n101 = Empty String/Path?(string/path=w374) -> (empty?=w375:bool)
            n102 = case shown="False" w375 {
              tunnel: w378 -> [w391 _]
              tunnel: w377 -> [w389 _]
              tunnel: w374 -> [w380 _]
              tunnel: [w381 _] -> w376
              frame False {
                n103 = call "_Compare Two Paths - Scalar.vi"("path2"=w380, "path1"=w389) -> ("relative path from 1 to 2"=w392:path)  [unwired: 1 in, 2 out]
                n104 = Build Path(base path=w391, name or relative path=w392) -> (appended path=w390:path)
                n105 = call <vilib>:"Check if File or Folder Exists.vi"("path"=w390) -> ("error out"=w386:errorcluster, "file or folder exists?"=w387:bool, "dup path"=w388:path)  [unwired: 8 in]
                n106 = case shown="True" w387 {
                  tunnel: w388 -> [w394 w398]
                  tunnel: [w394 w397] -> w385
                  tunnel: w386 -> [w393 w396]
                  tunnel: [w393 w395] -> w383
                  frame False {
                  }
                  frame True {
                    n107 = Delete(path (use dialog)=w398, error in=w396) -> (deleted path=w397:path, error out=w395:errorcluster)  [unwired: 3 in, 1 out]
                  }
                }
                n108 = Strip Path(path=w385) -> (stripped path=w384:path)  [unwired: 1 out]
                n109 = call <vilib>:"Create Directory Recursive.vi"("error in (no error)"=w383, "directory"=w384) -> ("error out"=w382:errorcluster)  [unwired: 3 in, 2 out]
                n110 = Move(source path=w380, error in=w382, 9:TRUE ("overwrite (F)"), 10:w385) -> (error out=w381:errorcluster)  [unwired: 1 in, 2 out]
              }
              frame True {
              }
            }
          }
          frame False {
            n111 = Empty String/Path?(string/path=w399) -> (empty?=w400:bool)
            n112 = case shown="False" w400 {
              tunnel: w403 -> [_ _]
              tunnel: w402 -> [_ _]
              tunnel: w399 -> [w405 _]
              tunnel: [w404 _] -> w401
              frame False {
                n113 = Delete(path (use dialog)=w405) -> (error out=w404:errorcluster)  [unwired: 4 in, 2 out]
              }
              frame True {
              }
            }
          }
        }
        n114 = call "Filter 1D Array_nevstop.vim"("items to filter"=w362, "array"=w363) -> ("filtered array"=w361:path[])  [unwired: 4 in, 1 out]
        n115 = Bundle By Name(cluster=w371, "Upload List"=w361, "Temp:UploadingFile"=path "") -> (w365:T6)
      }
      frame "FileSyncRoutine: Remove Empty Container Folder" {
        n116 = Unbundle By Name(w411) -> ("Configuration.MonitoringFolder"=w410:path)  [unwired: 1 out]
        n117 = String To Path(string=w409) -> (path=w408:path)
        n118 = Empty String/Path?(string/path=w408) -> (empty?=w407:bool)
        n119 = case shown="False" w407 {
          tunnel: w413 -> [w419 w441]
          tunnel: [w418 w441] -> w412
          tunnel: w410 -> [w417 _]
          tunnel: w408 -> [w416 _]
          frame False {
            n120 = while {
              tunnel: w417 -> [w426]
              shift-right: [w422] -> w418
              shift-left: w419 -> [w423]
              shift-right: [w421] -> _
              shift-left: w416 -> [w427]
              stop <- w420 stop-if-true
              n121 = Strip Path(path=w427) -> (stripped path=w421:path)  [unwired: 1 out]
              n122 = List Folder(path=w421, error in=w423) -> (path out=w428:path, filenames=w434:string[], folder names=w433:string[], error out=w425:errorcluster)  [unwired: 2 in]
              n123 = Empty Array?(array=w434) -> (empty?=w432:bool)
              n124 = Empty Array?(array=w433) -> (empty?=w431:bool)
              n125 = Not Equal?(x=w426, y=w421) -> (x != y?=w429:bool)
              n126 = And(x=w432, y=w431) -> (x .and. y?=w430:bool)
              n127 = And(x=w429, y=w430) -> (x .and. y?=w424:bool)
              n128 = case shown="False" w424 {
                tunnel: w428 -> [_ w440]
                tunnel: w425 -> [w436 w439]
                tunnel: [w436 w438] -> w422
                tunnel: [TRUE FALSE] -> w420
                frame False {
                }
                frame True {
                  n129 = Delete(path (use dialog)=w440, error in=w439) -> (error out=w438:errorcluster)  [unwired: 3 in, 2 out]
                }
              }
            }
          }
          frame True {
          }
        }
      }
    }
  }
